vi "Spline_Inter_Extrap.vi"(0 "Y calib points":dbl[](array[numeric]) format="%.3f", 1 "X calib points":dbl[](array[numeric]) format="%.3f", 2 "Calib constants":dbl[](array[numeric]) format="%.2f", 3 "Ch voltage":dbl format="%.4f") -> (5 "Output value":dbl format="%.3f", 7 "Error message":string)   [LabVIEW 2010]
uses:
  <vilib>/Analysis/NI_AALPro.lvlib
  <vilib>/Analysis/NI_AALBase.lvlib
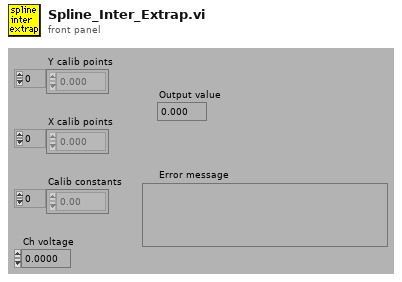
[diagram p1: front panel]
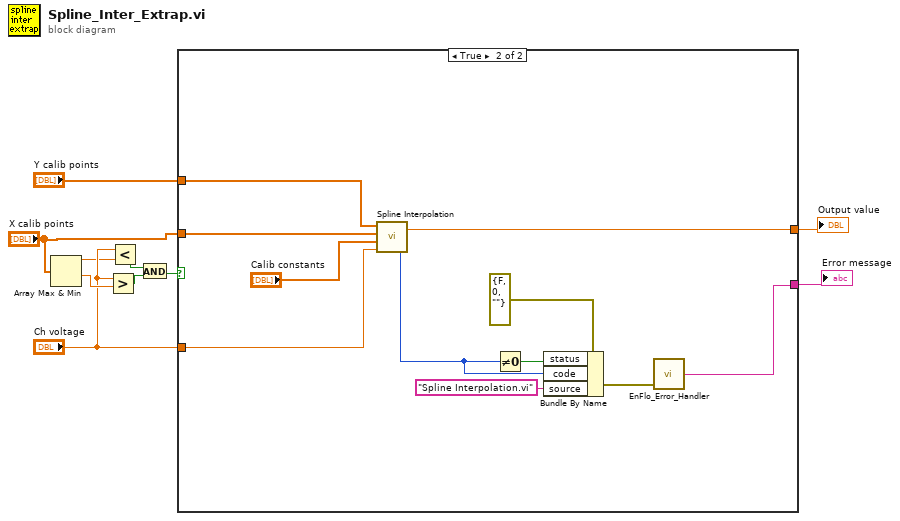
[diagram p0: block diagram]
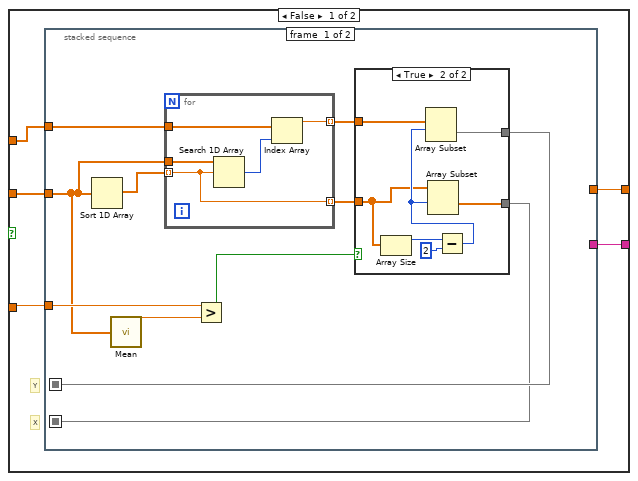
[diagram p2: hidden frame]
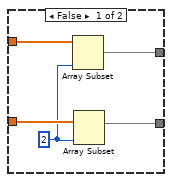
[diagram p3: hidden frame]
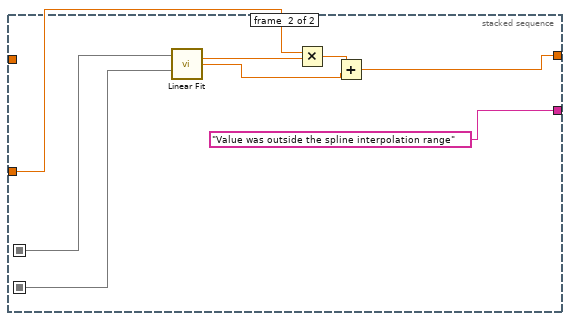
[diagram p4: hidden frame]
diagram:
  n1 = Array Max & Min(array="X calib points") -> (max value=w4:dbl, min value=w6:dbl)  [unwired: 2 out]
  n2 = Greater?(x="Ch voltage", y=w6) -> (0:w3:bool)
  n3 = Less?(x="Ch voltage", y=w4) -> (x < y?=w2:bool)
  n4 = And(x=w2, y=w3) -> (x .and. y?=w1:bool)
  n5 = case shown="True" w1 {
    tunnel: "Y calib points" -> [w14 w61]
    tunnel: "X calib points" -> [w15 w59]
    tunnel: "Ch voltage" -> [w13 w58]
    tunnel: [w12 w57] -> w9
    tunnel: [w11 w51] -> w8
    frame False {
      # "X"
      # "Y"
      n6 = stacked-sequence {
        seq-local: [w19 _] -> [_ w50]
        seq-local: [w18 _] -> [_ w49]
        tunnel: w15 -> [w17 _]
        tunnel: w14 -> [w24 _]
        tunnel: w13 -> [w22 w48]
        tunnel: [_ w44] -> w12
        tunnel: [_ "Value was outside the spline interpolation range"] -> w11
        frame #0 {
          n7 = Sort 1D Array(array=w17) -> (sorted array=w25:dbl[])
          n8 = call <vilib>:"Mean.vi"("X"=w17) -> ("mean"=w16:dbl)  [unwired: 1 out]
          n9 = for {
            tunnel: w17 -> [w42]
            tunnel: w25 -> [w38] mode=indexing
            tunnel: w24 -> [w40]
            tunnel: [w39] -> w23 mode=indexing
            tunnel: [w38] -> w20 mode=indexing
            n10 = Search 1D Array(1D array=w42, element=w38) -> (index of element=w41:i32)  [unwired: 1 out]
            n11 = Index Array(array=w40, index=w41) -> (element=w39:dbl)
          }
          n12 = Greater?(x=w22, y=w16) -> (0:w21:bool)
          n13 = case shown="True" w21 {
            tunnel: w23 -> [w30 w34]
            tunnel: w20 -> [w29 w33]
            tunnel: [w27 w32] -> w19
            tunnel: [w26 w31] -> w18
            frame False {
              w28 = 2 ("index")
              n14 = Array Subset(array=w30, length=w28) -> (w27:dbl[])  [unwired: 1 in]
              n15 = Array Subset(array=w29, length=w28) -> (w26:dbl[])  [unwired: 1 in]
            }
            frame True {
              n16 = Array Size(array=w33) -> (size(s)=w37:i32)
              n17 = Subtract(x=w37, y=2) -> (x-y=w35:i32)
              n18 = Array Subset(array=w34, index=w35) -> (w32:dbl[])  [unwired: 1 in]
              n19 = Array Subset(array=w33, index=w35) -> (w31:dbl[])  [unwired: 1 in]
            }
          }
        }
        frame #1 {
          n20 = call <vilib>:"Linear Fit.vi"("Y"=w50, "X"=w49) -> ("slope"=w47:dbl, "intercept"=w45:dbl)  [unwired: 4 in, 8 out]
          n21 = Multiply(x=w48, y=w47) -> (x*y=w46:dbl)
          n22 = Add(x=w46, y=w45) -> (x+y=w44:dbl)
        }
      }
    }
    frame True {
      n23 = call <vilib>:"Spline Interpolation.vi"("x value"=w58, "Interpolant"="Calib constants", "X"=w59, "Y"=w61) -> ("error"=w54:i32, "interpolation value"=w57:dbl)
      n24 = Not Equal To 0?(x=w54) -> (x != 0?=w55:bool)
      n25 = Bundle By Name(cluster=errorcluster {"status"=FALSE, "code"=0, "source"=""} ("error in (no error)"), "status"=w55, "code"=w54, "source"="Spline Interpolation.vi") -> (w52:errorcluster)
      n26 = call "EnFlo_Error_Handler.vi"("error in (no error)"=w52) -> ("SMS Message"=w51:string)  [unwired: 2 in, 2 out]
    }
  }
  "Error message" <- w8
  "Output value" <- w9
